vi "Calculate Electric Mobility.vi"(8 "error in (no error)":errorcluster, 11 "Particles in":refnum<class "Particle Properties.lvclass">) -> (0 "error out":errorcluster, 2 "Z":dbl, 3 "Particles out":refnum<class "Particle Properties.lvclass">)   [LabVIEW 2014, in "Particle Properties.lvclass"]
uses:
  Particle Properties.lvclass
  Particle Properties.lvclass/Particle Properties.ctl
  Accessors/Read Gas Ref.vi
  Accessors/Read D.vi
  Calculate Cc.vi
  Atmospheric/Atmospheric Constants.vi
  Atmospheric/Gas Properties/Gas Properties.lvclass
  Atmospheric/Atmospheric Library.lvlib
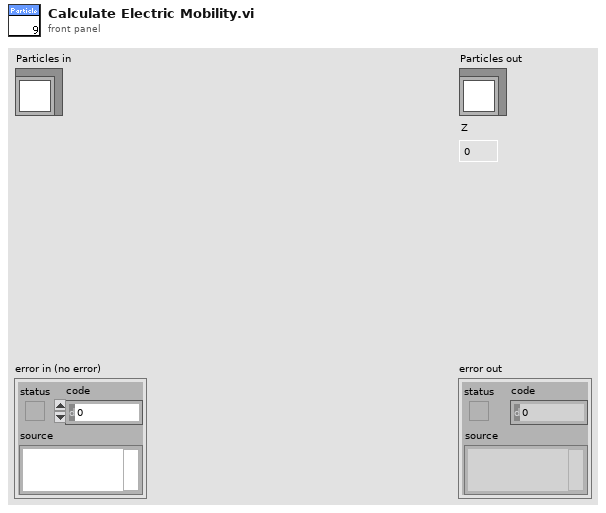
[diagram p1: front panel]
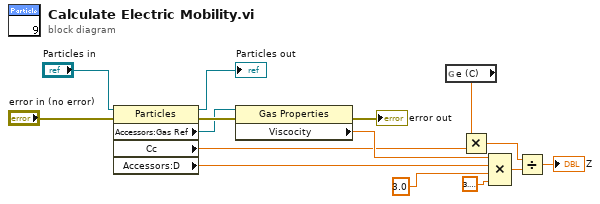
[diagram p0: block diagram]
diagram:
  n1 = property class="Particles"(reference="Particles in", error in="error in (no error)") -> (reference out=→"Particles out":refnum<class "Particle Properties.lvclass">, error out=w8:errorcluster, "Accessors:Gas Ref"=w1:refnum<data-value>, "Cc"=w2:dbl, "Accessors:D"=w14:dbl)
  n2 = property class="Gas Properties"(reference=w1, error in=w8) -> (error out=→"error out":errorcluster, "Viscocity"=w4:dbl)  [unwired: 1 out]
  n3 = global read "Atmospheric Constants.vi" "e (C)"() -> (w15:dbl)
  n4 = Multiply(x=w15, y=w2) -> (x*y=w11:dbl)
  n5 = Compound Arithmetic op=MULTIPLY(w4, w14, 3.0 ("value"), 3.141592653589793) -> (w12:dbl)
  n6 = Divide(x=w11, y=w12) -> (x/y=→"Z":dbl)
